vi "LV to ITX 2.2 1D multi.vi"(0 "Commands":string, 5 "filename":path, 7 "Notes":string, 8 "1D Arrays Names":string[](array[string]), 9 "1D Arrays":dbl[][](array[numeric]), 10 "2D Array name":string, 11 "2D Array":dbl[][](array[numeric])) -> ()   [LabVIEW 2011]
panel:
  out "String":string
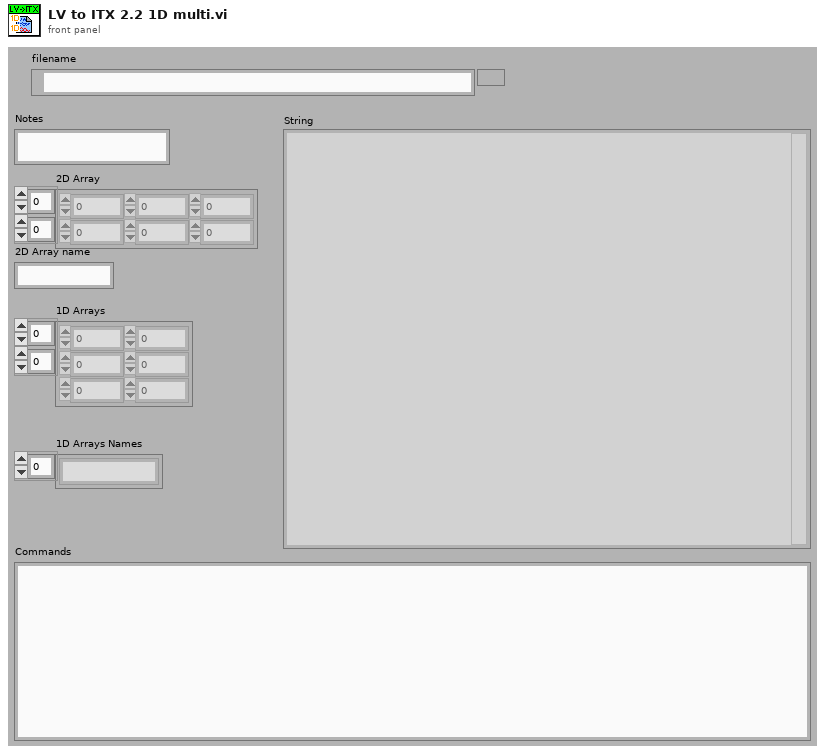
[diagram p1: front panel]
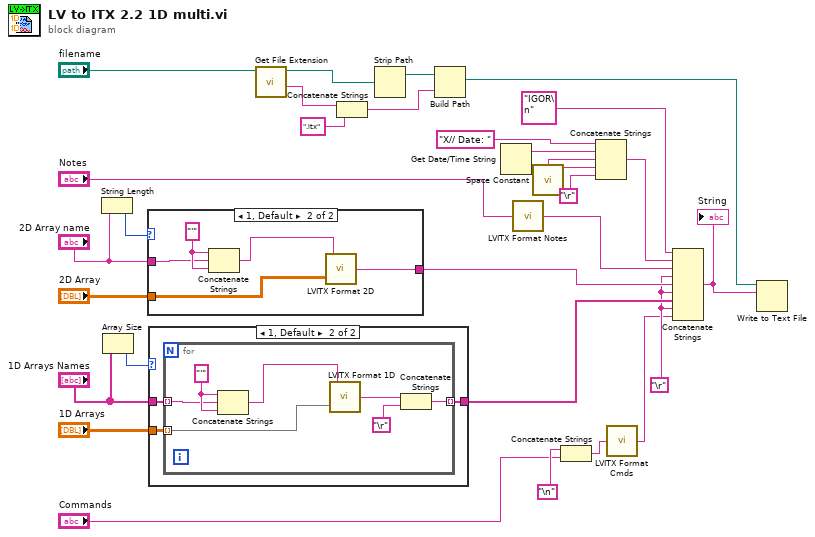
[diagram p0: block diagram]
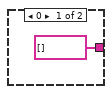
[diagram p2: hidden frame]
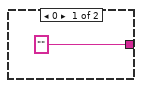
[diagram p3: hidden frame]
diagram:
  w11 = "\r"
  n1 = String Length(string="2D Array name") -> (length=w5:i32)
  n2 = Array Size(array="1D Arrays Names") -> (size(s)=w7:i32)
  n3 = case shown="1, Default" w5 {
    tunnel: ["" ("String") w35] -> w25
    tunnel: "2D Array name" -> [_ w33]
    tunnel: "2D Array" -> [_ w36]
    frame 0 {
    }
    frame 1, Default {
      w34 = "'"
      n4 = Concatenate Strings(w34, w33, w34) -> (w32:string)
      n5 = call "LVITX Format 2D.vi"("2D Array"=w36, "2D Array name"=w32) -> ("String"=w35:string)
    }
  }
  n6 = case shown="1, Default" w7 {
    tunnel: "1D Arrays Names" -> [_ w40]
    tunnel: "1D Arrays" -> [_ w39]
    tunnel: [string[] [] w38] -> w15
    frame 0 {
    }
    frame 1, Default {
      n7 = for {
        tunnel: [w47] -> w38 mode=indexing
        tunnel: w40 -> [w42] mode=indexing
        tunnel: w39 -> [w45] mode=indexing
        w43 = "'"
        n8 = Concatenate Strings(w43, w42, w43) -> (w41:string)
        n9 = call "LVITX Format 1D.vi"("X 1D Array"=w45, "X  Array name"=w41) -> ("String"=w44:string)
        n10 = Concatenate Strings(w44, "\r") -> (w47:string)
      }
    }
  }
  n11 = call <vilib>:"Get File Extension.vi"("file"="filename") -> ("filename without extension"=w22:string, "dup file"=w20:path)  [unwired: 1 in, 8 out]
  n12 = Concatenate Strings(w22, ".itx") -> (w18:string)
  n13 = Strip Path(path=w20) -> (stripped path=w19:path)  [unwired: 1 out]
  n14 = Build Path(base path=w19, name or relative path=w18) -> (appended path=w14:path)
  n15 = Get Date/Time String() -> (date string=w29:string, time string=w30:string)  [unwired: 3 out]
  n16 = call "LVITX Format Notes.vi"("Notes"="Notes") -> ("String"=w2:string)
  n17 = call <vilib>:"Space Constant.vi"() -> ("String"=w24:string)
  n18 = Concatenate Strings("\n", "Commands") -> (w4:string)
  n19 = Concatenate Strings("X// Date: " ("format string"), w29, w24, w30, "\r") -> (w28:string)
  n20 = call "LVITX Format Cmds.vi"("Commands"=w4) -> ("String"=w3:string)
  n21 = Concatenate Strings("IGOR\n", w28, w2, w11, w25, w11, w15, w11, w3) -> (w13:string)
  "String" <- w13
  n22 = Write to Text File(file (use dialog)=w14, text=w13) -> ()  [unwired: 1 in, 4 out]
